vi "Library Revision.vi"(8 "error in (no error)":errorcluster) -> (0 "error out":errorcluster, 2 "Library Revision":string)   [LabVIEW 2015, in "ZaberTSeries.lvlib"]
doc: "Retrieve the version number of this library."
uses:
  ZaberTSeries.lvlib
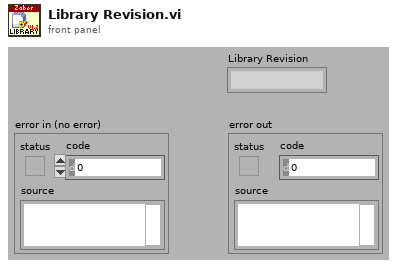
[diagram p1: front panel]
types:
  T1 = cluster{"Major":u16, "Minor":u16, "Fix":u16, "Build":u16}
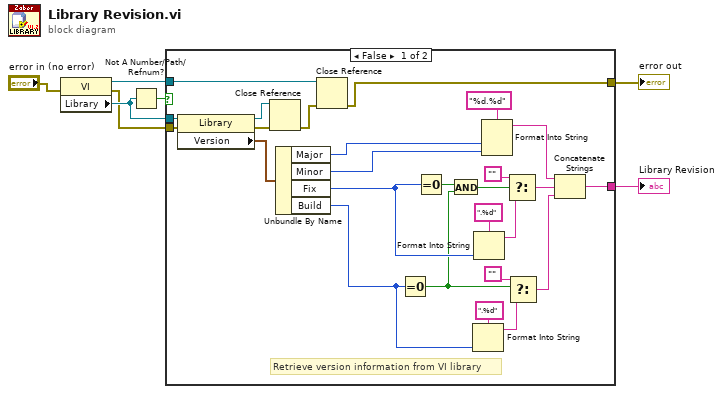
[diagram p0: block diagram]
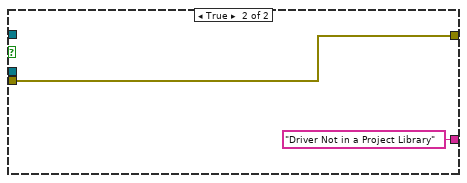
[diagram p2: hidden frame]
diagram:
  n1 = property class="VI"(error in="error in (no error)") -> (reference out=w1:refnum<vi>, error out=w2:errorcluster, "Library"=w3:refnum<vi>)  [unwired: 1 in]
  n2 = Not A Number/Path/Refnum?(number/path/refnum=w3) -> (NaN/Path/Refnum?=w4:bool)
  n3 = case shown="False" w4 {
    tunnel: w1 -> [w30 _]
    tunnel: w2 -> [w15 w35]
    tunnel: [w10 w35] -> w7
    tunnel: [w9 "Driver Not in a Project Library"] -> w5
    tunnel: w3 -> [w8 _]
    frame False {
      # "Retrieve version information from VI library"
      n4 = property class="Library"(reference=w8, error in=w15) -> (reference out=w32:refnum<vi>, error out=w33:errorcluster, "Version"=w29:T1)
      n5 = Close Reference(reference=w32, error in (no error)=w33) -> (error out=w31:errorcluster)
      n6 = Unbundle By Name(w29) -> ("Major"=w18:u16, "Minor"=w17:u16, "Fix"=w14:u16, "Build"=w16:u16)
      n7 = Close Reference(reference=w30, error in (no error)=w31) -> (error out=w10:errorcluster)
      n8 = Equal To 0?(x=w16) -> (x = 0?=w12:bool)
      n9 = Equal To 0?(x=w14) -> (x = 0?=w13:bool)
      n10 = And(x=w13, y=w12) -> (x .and. y?=w11:bool)
      n11 = Format Into String(format string=".%d", w16) -> (resulting string=w22:string)  [unwired: 2 in, 1 out]
      n12 = Format Into String(format string=".%d", w14) -> (resulting string=w26:string)  [unwired: 2 in, 1 out]
      n13 = Format Into String(format string="%d.%d", w18, w17) -> (resulting string=w24:string)  [unwired: 2 in, 1 out]
      n14 = Select(t="", s=w11, f=w26) -> (s? t:f=w23:string)
      n15 = Select(t="", s=w12, f=w22) -> (s? t:f=w19:string)
      n16 = Concatenate Strings(w24, w23, w19) -> (w9:string)
    }
    frame True {
    }
  }
  "error out" <- w7
  "Library Revision" <- w5
